vi "Get configuration chain.vi"(8 "error in (no error)":errorcluster, 11 "Cascade512IIBase in":refnum<class "DAQCascade512II.lvclass">) -> (0 "error out":errorcluster, 1 "class name":string[](array[string]), 2 "configuration chain":variant[](array[variant]), 3 "Cascade512IIBase out":refnum<class "DAQCascade512II.lvclass">)   [LabVIEW 2012, in "DAQCascade512II.lvclass"]
doc: "Returns an array of variants containing the configuration clusters of each class in the inheritance chain (lowest child class first), together with an array of all class names in the inheritance chain.\n\nFor classes without configuration cluster, the configuration chain contains empty variants."
uses:
  DAQCascade512II.lvclass
  <vilib>/Distrio/Murmex/Murmex/Murmex.lvclass
  DAQCascade512II.lvclass/DAQCascade512II.ctl
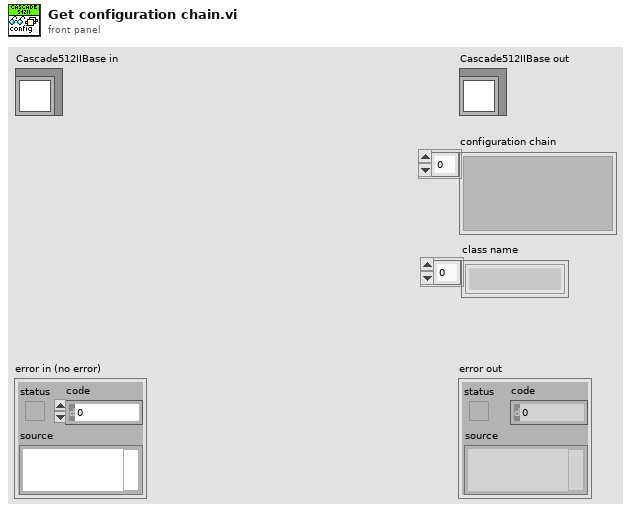
[diagram p1: front panel]
types:
  T1 = typedef "DAQCascade512II.lvclass/configuration cluster.ctl" = cluster{"Temperature":dbl, "Acquire / Focus Flag  of trigger":u32, "Number of Images fo Initializer":u32, "Data Type":u32, "Timing Mode of trigger ":u32, "Gain multiplication":dbl, "Fast ADC":bool}
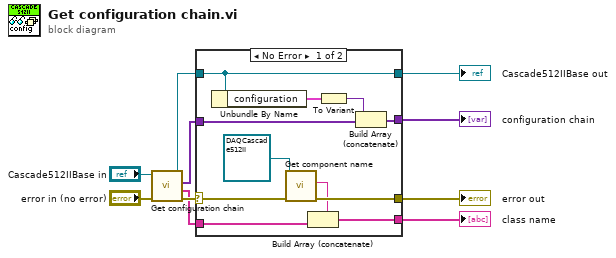
[diagram p0: block diagram]
diagram:
  n1 = call-parent "Get configuration chain.vi"("error in (no error)"="error in (no error)", "MurmexBase in"="Cascade512IIBase in") -> ("error out"=w8:errorcluster, "class name"=w6:string[], "configuration chain"=w4:variant[], "MurmexBase out"=w1:refnum<class "DAQCascade512II.lvclass">)  [unwired: 6 in]
  n2 = case shown="No Error" w8 {
    selector: w8 -> [w19 w25]
    tunnel: [w18 w25] -> w7
    tunnel: w6 -> [w16 w22]
    tunnel: [w15 w22] -> w5
    tunnel: w4 -> [w21 w24]
    tunnel: [w20 w24] -> w3
    tunnel: [w14 w23] -> w2
    tunnel: w1 -> [w14 w23]
    frame No Error {
      n3 = Unbundle By Name(w14) -> ("configuration"=w13:T1)
      n4 = call <vilib>:"Get component name.vi"("error in (no error)"=w19, "Murmex in"=refnum<class "DAQCascade512II.lvclass"> refnum ("DAQCascade512II")) -> ("error out"=w18:errorcluster, "component name"=w17:string)  [unwired: 7 in, 1 out]
      n5 = Build Array (concatenate)(w17, w16) -> (w15:string[])
      n6 = To Variant(anything=w13) -> (Variant=w12:variant)
      n7 = Build Array (concatenate)(w12, w21) -> (w20:variant[])
    }
    frame Error {
    }
  }
  "error out" <- w7
  "Cascade512IIBase out" <- w2
  "configuration chain" <- w3
  "class name" <- w5
